vi "FTW-CodeGen-OnResize2.vi"(0 "State In":T3 {"Width" format="%dpx"}, 5 "XRef":refnum<vi>, 7 "Bounds":T2, 9 "Mouse Mods":T1) -> (4 "State Out":T3 {"Width" format="%dpx"}, 6 "Reply":string[](array[string]))   [LabVIEW 2015, in "FTW-Dataflow-Burrow.xnode"]
uses:
  FTW-Dataflow-Burrow.xnode
  FTW-CodeGen-State.ctl
  framework/FTW-CodeGen-XNodeReplyType.ctl
panel:
  # "Inputs"
  # "Outputs"
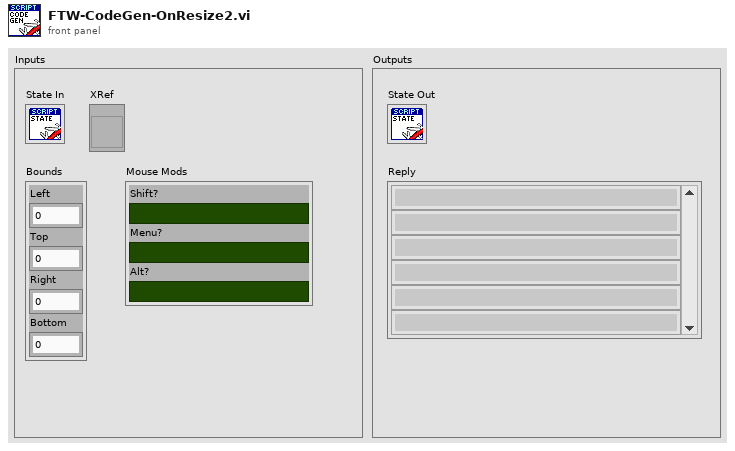
[diagram p1: front panel]
types:
  T1 = cluster{"Shift?":bool, "Menu?":bool, "Alt?":bool}
  T2 = cluster{"Left":i32, "Top":i32, "Right":i32, "Bottom":i32}
  T3 = typedef "FTW-Dataflow-Burrow.xnode/FTW-CodeGen-State.ctl" = cluster{"InputTerminals":cluster{"Wired?":bool, "ID":string, "DataName":string, "DataColor":u32, "Type":variant}[], "EnableTiming?":bool, "Width":i32}
  T4 = typedef "FTW-CodeGen-XNodeReplyType.ctl" = enum16{"NoReply", "ForceAdaptToInputs", "UpdateTerms", "GenCode", "GenCode+CosmeticUpdate"}
  T5 = cluster{"Wired?":bool, "ID":string, "DataName":string, "DataColor":u32, "Type":variant}[]
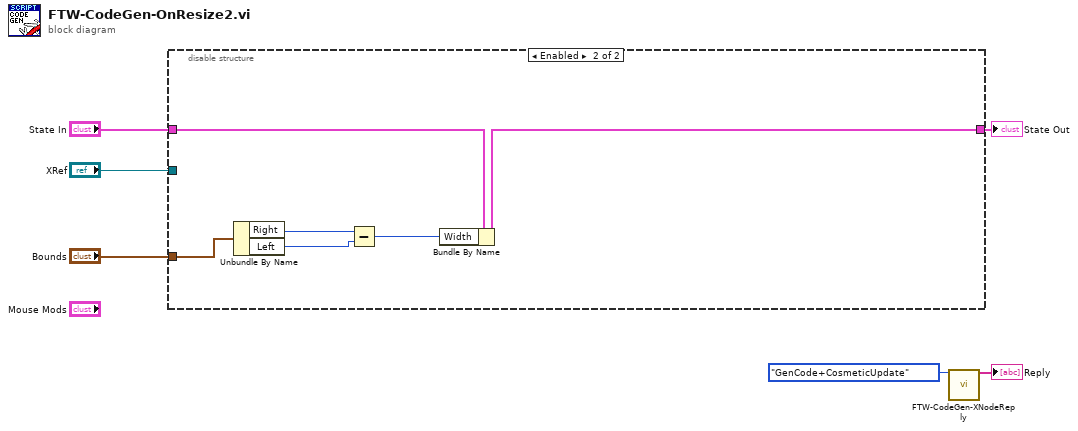
[diagram p0: block diagram]
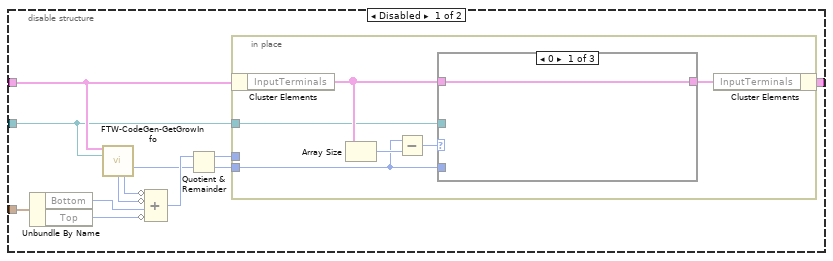
[diagram p2: hidden frame]
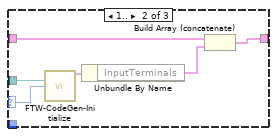
[diagram p3: hidden frame]
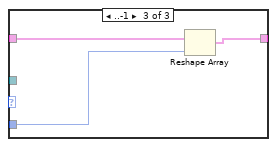
[diagram p4: hidden frame]
diagram:
  n1 = disable-structure shown="Enabled" {
    disable-tunnel: "Bounds" -> [w18 w39]
    disable-tunnel: "State In" -> [w11 w40]
    disable-tunnel: [w10 w36] -> w4
    disable-tunnel: "XRef" -> [w8 _]
    frame Disabled {
      n2 = Unbundle By Name(w18) -> ("Bottom"=w17:i32, "Top"=w16:i32)
      n3 = call "FTW-CodeGen-GetGrowInfo.vi"("State In"=w11, "XRef"=w8) -> ("Terminal Height"=w12:i32, "Bottom Banner Height"=w14:i32, "Total Top Banner Height"=w15:i32)  [unwired: 5 in, 6 out]
      n4 = Compound Arithmetic op=ADD(invert w15, invert w14, w17, invert w16) -> (w13:i32)
      n5 = Quotient & Remainder(x=w13, y=w12) -> (x-y*floor(x/y)=w7:i32, floor(x/y)=w9:i32)
      n6 = in-place {
        in-place-border: w9 -> [w21]
        in-place-border: w8 -> [w19]
        in-place-border: w7 -> [_]
        n7 = in-place-cluster #1(w11) -> ("InputTerminals"=w23:T5)
        n8 = Array Size(array=w23) -> (size(s)=w22:i32)
        n9 = Subtract(x=w21, y=w22) -> (x-y=w20:i32)
        n10 = case shown="0" w20 {
          selector: w20 -> [_ w30 _]
          tunnel: [w25 w28 w34] -> w24
          tunnel: w23 -> [w25 w31 w33]
          tunnel: w21 -> [_ _ w32]
          tunnel: w19 -> [_ w29 _]
          frame 0 {
          }
          frame 1.. {
            n11 = call "FTW-CodeGen-Initialize.vi"("XRef"=w29, "Items"=w30) -> ("State Out"=w27:T3)  [unwired: 13 in]
            n12 = Unbundle By Name(w27) -> ("InputTerminals"=w26:T5)
            n13 = Build Array (concatenate)(w31, w26) -> (w28:T5)
          }
          frame ..-1 {
            n14 = Reshape Array(w33, w32) -> (w34:T5)
          }
        }
        n15 = in-place-cluster #1("InputTerminals"=w24) -> (w10:T3)
      }
    }
    frame Enabled {
      n16 = Unbundle By Name(w39) -> ("Right"=w38:i32, "Left"=w37:i32)
      n17 = Subtract(x=w38, y=w37) -> (x-y=w35:i32)
      n18 = Bundle By Name(cluster=w40, "Width"=w35) -> (w36:T3)
    }
  }
  "State Out" <- w4
  n19 = call "FTW-CodeGen-XNodeReply.vi"("XNode Reply Type"=FTW-CodeGen-XNodeReplyType."GenCode+CosmeticUpdate") -> ("Reply"=→"Reply":string[])  [unwired: 14 in]
